vi "Fit complex bg one.vi"(7 "Bounds":T1={"parameter minimum"=[1.0, 1.0, 0.01, -0.1, -5.0, -5.0], "parameter maximum"=[20000000.0, 200.0, 100.0, 6.3, 5.0, 5.0]}, 8 "Error In":errorcluster, 9 "Initial parameters":dbl[](array[numeric])=[188.484, 0.01, 0.00126452, 2.4, 1.1376494443646765, -0.8104040332703796], 10 "Z":cdb[](array[numeric]), 11 "X":dbl[](array[numeric])) -> (0 "Error Out":errorcluster, 2 "Plot":cluster{"X":dbl[], "Array":dbl[]}[](array[cluster]), 3 "best fit parameters":dbl[](array[numeric]))   [LabVIEW 2016]
uses:
  <vilib>/gmath/NumericalOptimization/Nonlinear Curve Fit LM.vi
  <vilib>/gmath/NI_Gmath.lvlib
  <vilib>/gmath/NumericalOptimization/Nonlinear Curve Fit LM bound.vi
panel:
  out "residue":dbl
  out "Weight":dbl[](graph)
  out "number of function calls":i32
  in  "termination":cluster{"max iteration":i32, "tolerance":dbl}={"max iteration"=2000, "tolerance"=1e-08}
  out "Fit":cluster{"X":dbl[], "best nonlinear fit":dbl[]}[](graph)
  # "F0\nG\nA\nP\nX\nY"
  # "F0\nG\nA\nP\nX\nY"
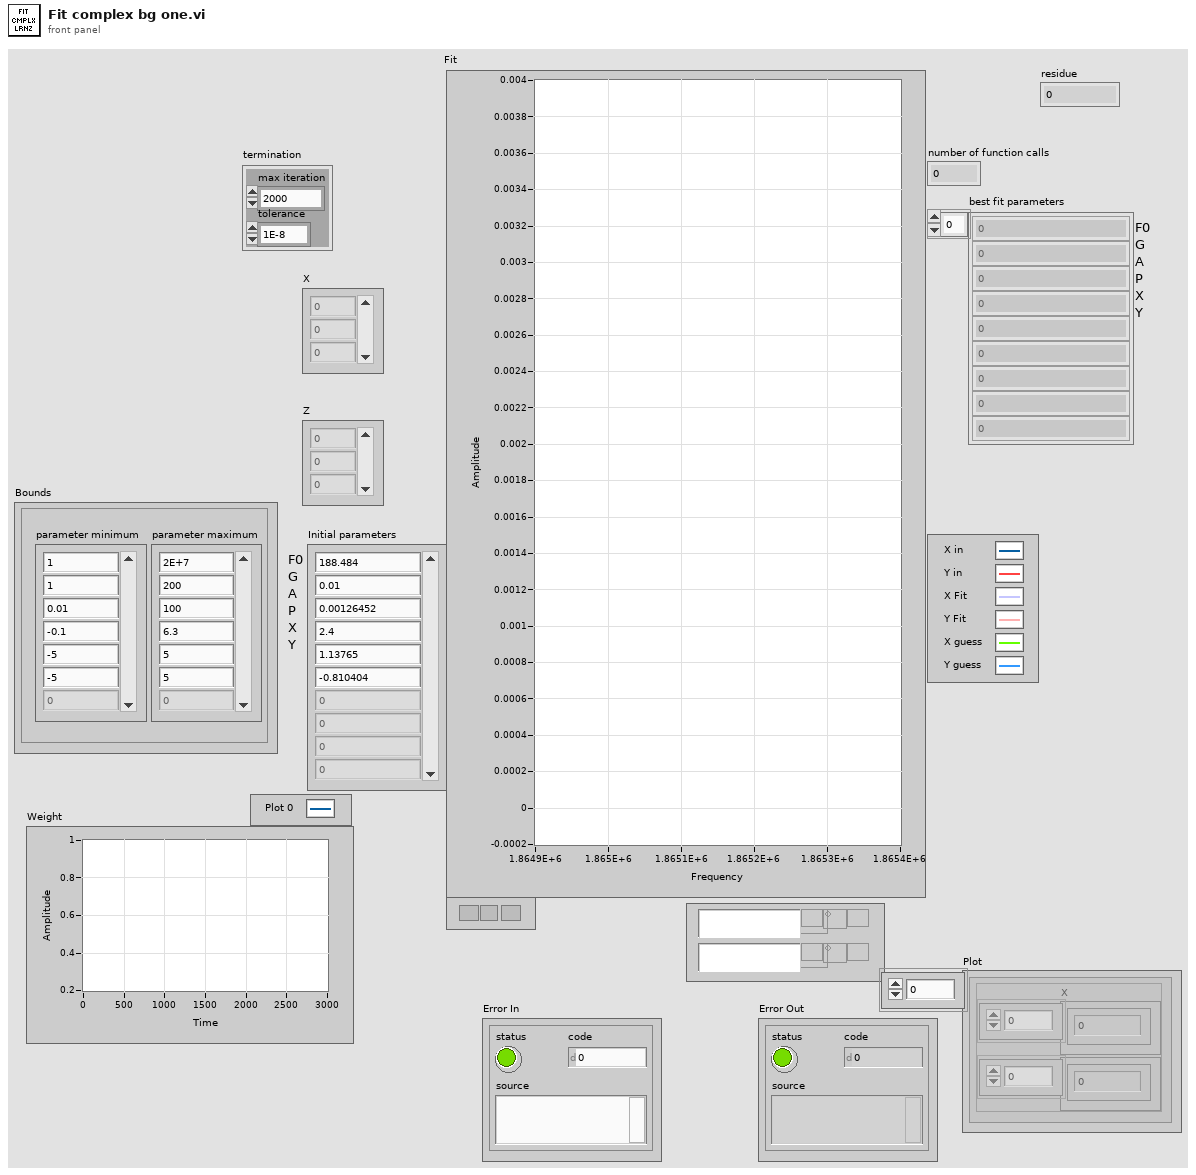
[diagram p1: front panel]
types:
  T1 = cluster{"parameter minimum":dbl[], "parameter maximum":dbl[]}
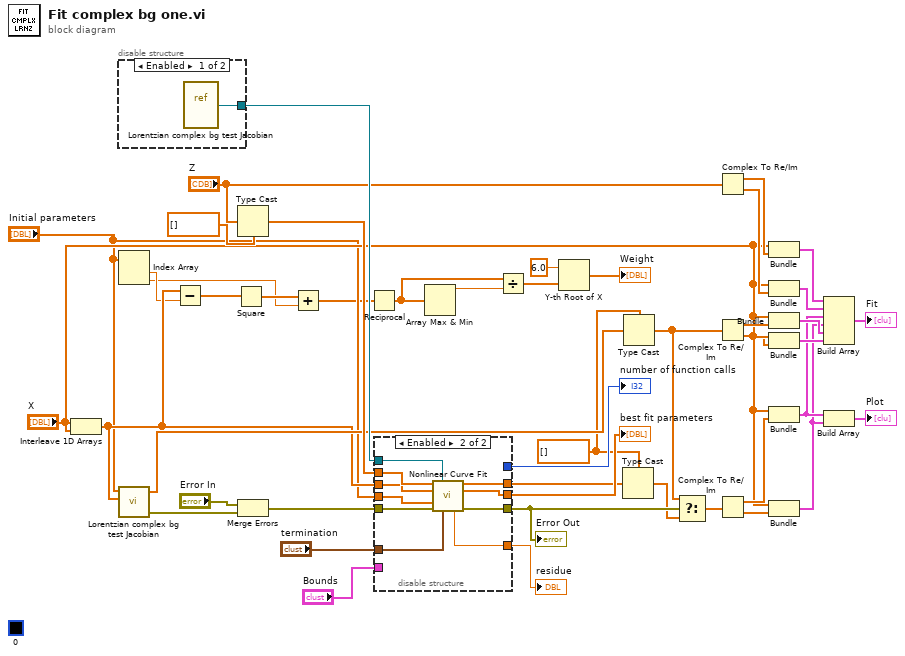
[diagram p0: block diagram]
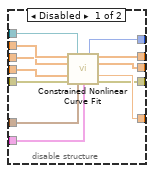
[diagram p2: hidden frame]
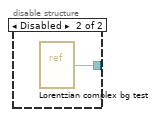
[diagram p3: hidden frame]
diagram:
  (unwired) u32 0 ("Color Box")
  w29 = cdb[] []
  n1 = Interleave 1D Arrays("X", "X") -> (w24:dbl[])
  n2 = disable-structure shown="Enabled" {
    disable-tunnel: [w47 w48] -> w46
    frame Enabled {
      n3 = vi-ref "Lorentzian complex bg test Jacobian.vi"() -> (w47:refnum<vi>)
    }
    frame Disabled {
      n4 = vi-ref "Lorentzian complex bg test.vi"() -> (w48:refnum<vi>)
    }
  }
  n5 = Index Array(array="Initial parameters") -> (element #1=w22:dbl, element #2=w19:dbl)  [unwired: 2 in]
  n6 = call "Lorentzian complex bg test Jacobian.vi"("X"=w24, "a"="Initial parameters") -> ("error out"=w9:errorcluster, "f(X,a)"=w30:dbl[])  [unwired: 2 in, 1 out]
  n7 = Subtract(x=w24, y=w22) -> (x-y=w21:dbl[])
  n8 = Square(x=w21) -> (x^2=w20:dbl[])
  n9 = Type Cast(type=dbl[] [], x="Z") -> (*(type *) &x=w40:dbl[])
  n10 = Merge Errors("Error In", w9) -> (w8:errorcluster)
  n11 = Add(x=w20, y=w19) -> (x+y=w18:dbl[])
  n12 = Reciprocal(x=w18) -> (1/x=w17:dbl[])
  n13 = disable-structure shown="Enabled" {
    disable-tunnel: w46 -> [w60 w70]
    disable-tunnel: "termination" -> [w59 w64]
    disable-tunnel: [w58 _] -> w43
    disable-tunnel: [w57 w62] -> w42
    disable-tunnel: w40 -> [w56 w69]
    disable-tunnel: [w55 w61] -> w38
    disable-tunnel: w24 -> [w54 w68]
    disable-tunnel: "Initial parameters" -> [w53 w67]
    disable-tunnel: "Bounds" -> [w52 _]
    disable-tunnel: [w51 w63] -> w14
    disable-tunnel: w8 -> [w50 w66]
    disable-tunnel: [w49 w65] -> w4
    frame Disabled {
      n14 = call-poly <vilib>:"Constrained Nonlinear Curve Fit.vi"("Y"=w56, "f(x,a)"=w60, "X"=w54, "initial parameters"=w53, "error in (no error)"=w50, "termination"=w59, "parameter bounds"=w52) -> ("number of function calls"=w58:i32, "best nonlinear fit"=w55:dbl[], "best fit parameters"=w57:dbl[], "residue"=w51:dbl, "error out"=w49:errorcluster)  [unwired: 3 in, 1 out]
    }
    frame Enabled {
      n15 = call-poly <vilib>:"Nonlinear Curve Fit.vi"("Y"=w69, "f(x,a)"=w70, "X"=w68, "initial parameters"=w67, "error in (no error)"=w66, "termination"=w64) -> ("best nonlinear fit"=w61:dbl[], "best fit parameters"=w62:dbl[], "residue"=w63:dbl, "error out"=w65:errorcluster)  [unwired: 4 in, 2 out]
    }
  }
  "number of function calls" <- w43
  "best fit parameters" <- w42
  "residue" <- w14
  "Error Out" <- w4
  n16 = Array Max & Min(array=w17) -> (max value=w16:dbl)  [unwired: 3 out]
  n17 = Divide(x=w17, y=w16) -> (x/y=w13:dbl[])
  n18 = Y-th Root of X(1:w13, 2:6.0) -> (0:→"Weight":dbl[])
  n19 = Type Cast(type=w29, x=w38) -> (*(type *) &x=w2:cdb[])
  n20 = Type Cast(type=w29, x=w30) -> (*(type *) &x=w3:cdb[])
  n21 = Select(t=w3, s=w4, f=w2) -> (s? t:f=w1:cdb[])
  n22 = Complex To Re/Im(x + iy="Z") -> (x=w36:dbl[], y=w35:dbl[])
  n23 = Complex To Re/Im(x + iy=w3) -> (x=w28:dbl[], y=w26:dbl[])
  n24 = Complex To Re/Im(x + iy=w1) -> (x=w31:dbl[], y=w32:dbl[])
  n25 = Bundle("X"="X", w36) -> (w34:cluster{"X":dbl[], dbl[]})  [unwired: 1 in]
  n26 = Bundle("X"="X", w35) -> (w33:cluster{"X":dbl[], dbl[]})  [unwired: 1 in]
  n27 = Bundle("X"="X", w28) -> (w41:cluster{"X":dbl[], dbl[]})  [unwired: 1 in]
  n28 = Bundle("X"="X", w26) -> (w25:cluster{"X":dbl[], dbl[]})  [unwired: 1 in]
  n29 = Bundle("X"="X", w31) -> (w7:cluster{"X":dbl[], dbl[]})  [unwired: 1 in]
  n30 = Bundle("X"="X", w32) -> (w6:cluster{"X":dbl[], dbl[]})  [unwired: 1 in]
  n31 = Build Array(w34, w33, w7, w6, w41, w25) -> (→"Fit":cluster{"X":dbl[], dbl[]}[])
  n32 = Build Array(w7, w6) -> (→"Plot":cluster{"X":dbl[], dbl[]}[])
